vi "KnobType.vi"(9 "Knob in":refnum<class "Knob.lvclass">) -> (3 "Knob out":refnum<class "Knob.lvclass">, 4 "Knob type":T1)   [LabVIEW 2014, in "Raspberry Pi Compatible Compiler for LabVIEW.lvlib" / "Knob.lvclass"]
uses:
  Knob.lvclass
  KnobTypesTD.ctl
  Control/Control.lvclass/Control.ctl
  Control/Control.lvclass
  Raspberry Pi Compatible Compiler for LabVIEW.lvlib
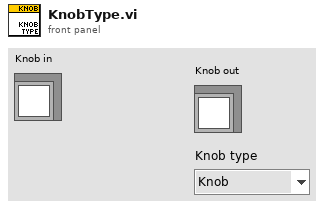
[diagram p1: front panel]
types:
  T1 = typedef "Raspberry Pi Compatible Compiler for LabVIEW.lvlib/KnobTypesTD.ctl" = enum16{"Knob", "Dial", "Meter", "Gauge"}
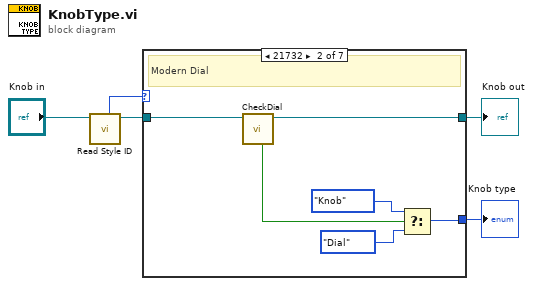
[diagram p0: block diagram]
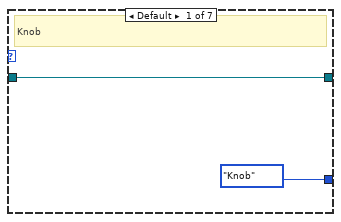
[diagram p2: hidden frame]
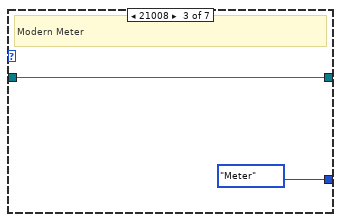
[diagram p3: hidden frame]
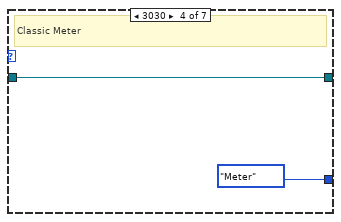
[diagram p4: hidden frame]
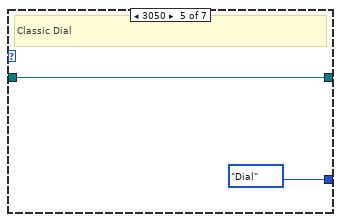
[diagram p5: hidden frame]
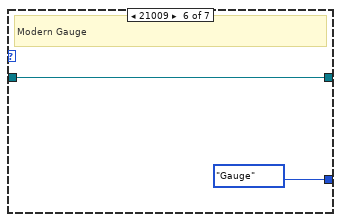
[diagram p6: hidden frame]
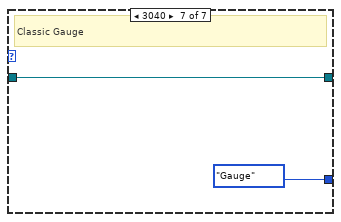
[diagram p7: hidden frame]
diagram:
  n1 = call "Read Style ID.vi"("Control in"="Knob in") -> ("Control out"=w3:refnum<class "Knob.lvclass">, "Style ID"=w4:u32)  [unwired: 7 in]
  n2 = case shown="21732" w4 {
    tunnel: w3 -> [w6 w13 w14 w16 w18 w20 w22]
    tunnel: [KnobTypesTD."Knob" ("Knob type") w11 KnobTypesTD."Meter" ("Knob type") KnobTypesTD."Meter" ("Knob type") KnobTypesTD."Dial" ("Knob type") KnobTypesTD."Gauge" ("Knob type") KnobTypesTD."Gauge" ("Knob type")] -> w2
    tunnel: [w6 w12 w14 w16 w18 w20 w22] -> w1
    frame Default {
      # "Knob"
    }
    frame 21732 {
      # "Modern Dial"
      n3 = call "CheckDial.vi"("Knob in"=w13) -> ("Knob out"=w12:refnum<class "Knob.lvclass">, "Knob"=w10:bool)  [unwired: 5 in, 2 out]
      n4 = Select(t=KnobTypesTD."Knob" ("Knob type"), s=w10, f=KnobTypesTD."Dial" ("Knob type")) -> (s? t:f=w11:T1)
    }
    frame 21008 {
      # "Modern Meter"
    }
    frame 3030 {
      # "Classic Meter"
    }
    frame 3050 {
      # "Classic Dial"
    }
    frame 21009 {
      # "Modern Gauge"
    }
    frame 3040 {
      # "Classic Gauge"
    }
  }
  "Knob out" <- w1
  "Knob type" <- w2
